vi "Credit.vi"(8 "error in (no error)":errorcluster, 10 "Monedas":T1, 11 "Dinero in":refnum<class "Dinero.lvclass">) -> (0 "error out":errorcluster, 3 "Dinero out":refnum<class "Dinero.lvclass">)   [LabVIEW 2020, in "Dinero.lvlib" / "Dinero.lvclass"]
uses:
  Dinero.lvclass
  C:/Program Files (x86)/National Instruments/LabVIEW 2020/vi.lib/ActorFramework/Actor/Actor.lvclass
  <vilib>/ActorFramework/Actor/Actor.lvclass/Actor.ctl
  Dinero.lvclass/Dinero.ctl
  User Interface Messages/Credit manage Msg/Credit manage Msg.lvclass/Credit manage Msg.ctl
  <vilib>/ActorFramework/Message Enqueuer/Message Enqueuer.lvclass/Message Enqueuer.ctl
  <vilib>/ActorFramework/Message Enqueuer/Enqueue.vi
  User Interface Messages/Credit manage Msg/Credit manage Msg.lvclass
  C:/Program Files (x86)/National Instruments/LabVIEW 2020/vi.lib/ActorFramework/Message/Message.lvclass
  <vilib>/ActorFramework/Message Priority Queue/Priority Enqueue.vi
  <vilib>/ActorFramework/Actor/Actor.lvclass
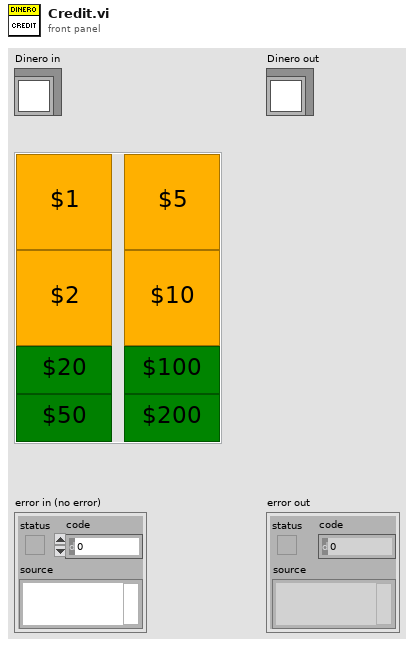
[diagram p1: front panel]
types:
  T1 = cluster{"Moneda 1":bool, "Moneda 2":bool, "Moneda 5":bool, "Moneda 10":bool, "Billete 20":bool, "Billete 50":bool, "Billete 100":bool, "Billete 200":bool}
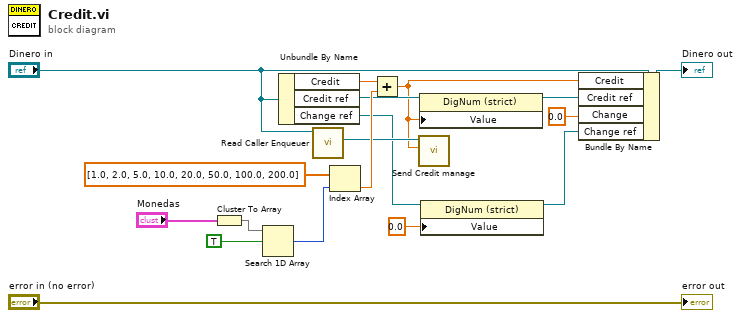
[diagram p0: block diagram]
diagram:
  n1 = Cluster To Array(cluster="Monedas") -> (array=w16:bool[])
  n2 = Search 1D Array(1D array=w16, element=TRUE) -> (index of element=w12:i32)  [unwired: 1 in]
  n3 = Unbundle By Name("Dinero in") -> ("Credit"=w10:dbl, "Credit ref"=w9:refnum<vi>, "Change ref"=w4:refnum<vi>)
  n4 = call <vilib>:"Read Caller Enqueuer.vi"("Actor"="Dinero in") -> ("Caller Enqueuer"=w6:refnum<class "Message Enqueuer.lvclass">)  [unwired: 10 in]
  n5 = Index Array(array=dbl[] [1.0, 2.0, 5.0, 10.0, 20.0, 50.0, 100.0, 200.0], index=w12) -> (element=w11:dbl)
  n6 = Add(x=w10, y=w11) -> (x+y=w5:dbl)
  n7 = call "Send Credit manage.vi"("Credit"=w5, "Message Enqueuer"=w6) -> ()  [unwired: 8 in, 2 out]
  n8 = property class="DigNum (strict)"(reference=w9, "Value"=w5) -> (reference out=w8:refnum<vi>)  [unwired: 1 in, 1 out]
  n9 = property class="DigNum (strict)"(reference=w4, "Value"=0.0) -> (reference out=w1:refnum<vi>)  [unwired: 1 in, 1 out]
  n10 = Bundle By Name(cluster="Dinero in", "Credit"=w5, "Credit ref"=w8, "Change"=0.0, "Change ref"=w1) -> (→"Dinero out":refnum<class "Dinero.lvclass">)
  "error out" <- "error in (no error)"
